vi "FRIC_navX_Internal_SPI_ProcessingLoop.vi"(7 "Device Number":T2, 11 "Rate (4Hz-200Hz)":u8=50 min=4 max=200) -> ()   [LabVIEW 2016]
doc: "This navX VI handles the reading/writing for the navX. All of the good stuff is in here.\nTHIS VI SHOULD NOT BE CALLED BY THE USER!"
uses:
  <vilib>/Rock Robotics/SystemInterfaces/i2clib/i2c_bus.ctl
  TypeDefs/Z900_navX_ProtocolTypeDef.ctl
  navX Library v2.lvlib
  TypeDefs/FRIC_navX_ProcessingLoopStatesTypeDef_I2C.ctl
  TypeDefs/Z900_navX_IntegrationControlRegisters.ctl
  TypeDefs/Z900_navX_ActionTypeDef.ctl
  TypeDefs/Z900_navX_NotifyPacketTypeDef.ctl
  TypeDefs/FRIC_navX_I2C Process Loop TypeDef.ctl
  TypeDefs/Flags/Z900_navX_Flags_CapabilityTypeDef.ctl
  TypeDefs/Z900_navX_DeviceRegisters.ctl
  <vilib>/Rock Robotics/SystemInterfaces/spilib/spi_bus.ctl
  <vilib>/Rock Robotics/WPI/SPI/WPI_SPIDevRef.ctl
  <vilib>/Rock Robotics/WPI/SerialPort/WPI_SerialPortRef.ctl
  TypeDefs/Z900_navX_SerialStreamTypeDef.ctl
  TypeDefs/FRIC_navX_DeviceNumbersTypeDef.ctl
  <vilib>/Rock Robotics/WPI/SerialPort/WPI_SerialPort.ctl
  <vilib>/Platform/TimedLoop/XDataNode/XDataNode.xnode
  <vilib>/Platform/TimedLoop/XDataNode/nitl_modes.ctl
  <vilib>/Platform/TimedLoop/XDataNode/XDNodeRunTimeDep.lvlib
  <vilib>/Platform/TimedLoop/XDataNode/wakeup.ctl
  <vilib>/Platform/TimedLoop/XDataNode/timing_clust.ctl
  <vilib>/ptbypt/NI_PtbyPt.lvlib
  TypeDefs/Z900_navX_DeviceTypeDef.ctl
panel:
  in  "Tab Control":enum32{"Page 1", "Page 2"}(tab)
  in  "Halt":bool
  out "Connected":bool
  in  "SPI Bus":T1=enum."SPI MXP"
  in  "Clock Rate (Hz)":dbl=2000000.0 format="%_6f"
  out "error":errorcluster
  out "Delay":dbl
  out "Loop Time":dbl format="%0.2f"
  out "Loop dt":i64
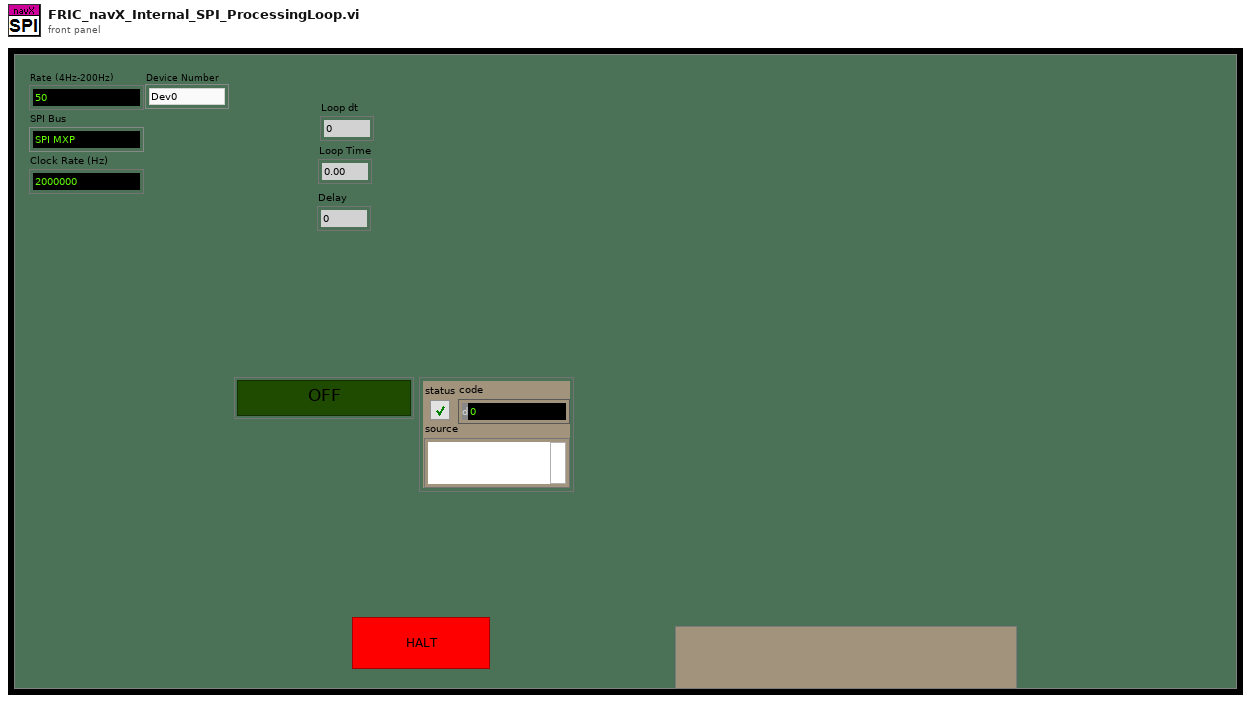
[diagram p1: front panel]
types:
  T1 = typedef "spi_bus.ctl" = enum16{"SPI On-Board, CS0", "SPI On-Board, CS1", "SPI On-Board, CS2", "SPI On-Board, CS3", "SPI MXP", "Invalid"}
  T2 = typedef "FRIC_navX_DeviceNumbersTypeDef.ctl" = enum16{"Dev0", "Dev1", "Dev2", "Dev3"}
  T3 = typedef "FRIC_navX_I2C Process Loop TypeDef.ctl" = cluster{"State Array":T4[], "error":errorcluster, "FPGA Cluster":cluster{"Last Valid FPGA Time":dbl, "Error Count":i32, "Initialized":bool}, "Device Info":T5, "I2CDevRef":cluster{"DevStatus":errorcluster, "Device Address":u8, "Handle":i32, "I2C Bus":T7}, "Registry":u8[], "Command Array":T8[], "Connected?":bool, "navX Device Memory Size":i32, "notification":T9, "Memory Size Set":bool, "SPIDevRef":T11, "navX Serial Open":cluster{"Stream Type":T12, "Serial Port":T13}, "SerialPortRef":T14, "Serial Read Buffer":string, "Serial Write Buffer":string[], "Device Number":T2, "navX SPI Open":cluster{"SPI Bus":T1, "Clock Rate (Hz)":dbl}, "Loop dt":i64, "current time":timestamp, "Loop Time":i64}
  T4 = typedef "FRIC_navX_ProcessingLoopStatesTypeDef_I2C.ctl" = enum16{"Process", "INI", "Check Packets Valid", "Close", "Flush Serial", "Generate Command", "Last Packet Valid", "Open", "Read", "Reset Serial", "Set Termination Char", "Update AE", "Wait", "Write", "Exit"}
  T5 = typedef "navX Library v2.lvlib/Z900_navX_DeviceTypeDef.ctl" = cluster{"Interface":cluster{"Protocol":T6, "Update Rate (4Hz-100Hz)":u8, "navX Open TypeDef":variant}, "Notify Packet":refnum<notifier>, "Loop VI Refnum":refnum<vi>, "Ready to Close Occurrence Refnum":refnum<k4>}
  T6 = typedef "navX Library v2.lvlib/Z900_navX_ProtocolTypeDef.ctl" = enum16{"SERIAL", "I2C", "SPI"}
  T7 = typedef "i2c_bus.ctl" = enum16{"I2C On-Board", "I2C MXP", "Invalid"}
  T8 = typedef "navX Library v2.lvlib/Z900_navX_IntegrationControlRegisters.ctl" = u8
  T9 = typedef "navX Library v2.lvlib/Z900_navX_NotifyPacketTypeDef.ctl" = cluster{"navX Action":T10, "Data":variant}
  T10 = typedef "navX Library v2.lvlib/Z900_navX_ActionTypeDef.ctl" = enum16{"None", "Halt", "Update Serial Protocol", "Zero-Yaw", "Zero-Displacement", "Zero-Velocity"}
  T11 = typedef "WPI_SPIDevRef.ctl" = cluster{"DevStatus":errorcluster, "Handle":i32, "SPI Bus":T1}
  T12 = typedef "navX Library v2.lvlib/Z900_navX_SerialStreamTypeDef.ctl" = enum16{"YRPH", "Quaterinons", "Gyro/Raw", "AHRS", "AHRSAndPositioning"}
  T13 = typedef "WPI_SerialPort.ctl" = enum16{"Onboard RS-232", "MXP TTL", "USB 1", "USB 2"}
  T14 = typedef "WPI_SerialPortRef.ctl" = cluster{"DevStatus":errorcluster, "Serial Port Name":refnum<visa-resource-name>}
  T15 = typedef "XDNodeRunTimeDep.lvlib/timing_clust.ctl" = cluster{"Expected End [f-1]":u64, "Actual End [f-1]":u64, "Finished Late? [f-1]":bool, "Expected End [i-1]":u64, "Actual End [i-1]":u64, "Finished Late? [i-1]":bool, "Expected Start [i]":u64, "Actual Start [i]":u64, "Expected Start [f]":u64, "Actual Start [f]":u64, "Source Name":string, "Structure Name":string, "Period":i64, "Deadline":i64, "Offset":i64, "Start":i64, "Priority":i32, "Timeout":i32, "Mode":T16, "Wakeup Reason":T17, "Error":errorcluster, "Source Type":string, "Secondary Source Type":string, "Global End Time":u64, "Global Start Time":u64, "Frame Duration":u64, "Iteration Duration":u64, "Assigned CPU":i32, "I/O Scan Engine Mode":u32}
  T16 = typedef "XDNodeRunTimeDep.lvlib/nitl_modes.ctl" = enum32{"No Change", "Process missed periods, maintain original phase", "Discard missed periods, maintain original phase", "Process missed periods, ignore original phase", "Discard missed periods, ignore original phase"}
  T17 = typedef "XDNodeRunTimeDep.lvlib/wakeup.ctl" = enum32{"Normal", "Aborted", "Asynchronous wakeup", "Timing source error", "Timed loop error", "Timeout"}
  T18 = typedef "Z900_navX_ActionTypeDef.ctl" = enum16{"None", "Halt", "Normal Read", "Update Serial Protocol", "Update Rate Htz", "Zero-Yaw", "Zero-Displacement", "Zero-Velocity"}
  T19 = typedef "navX Library v2.lvlib/Z900_navX_DeviceRegisters.ctl" = u8
  T20 = typedef "navX Library v2.lvlib/Z900_navX_Flags_CapabilityTypeDef.ctl" = u16
  T21 = cluster{"Last Valid FPGA Time":dbl, "Error Count":i32, "Initialized":bool}
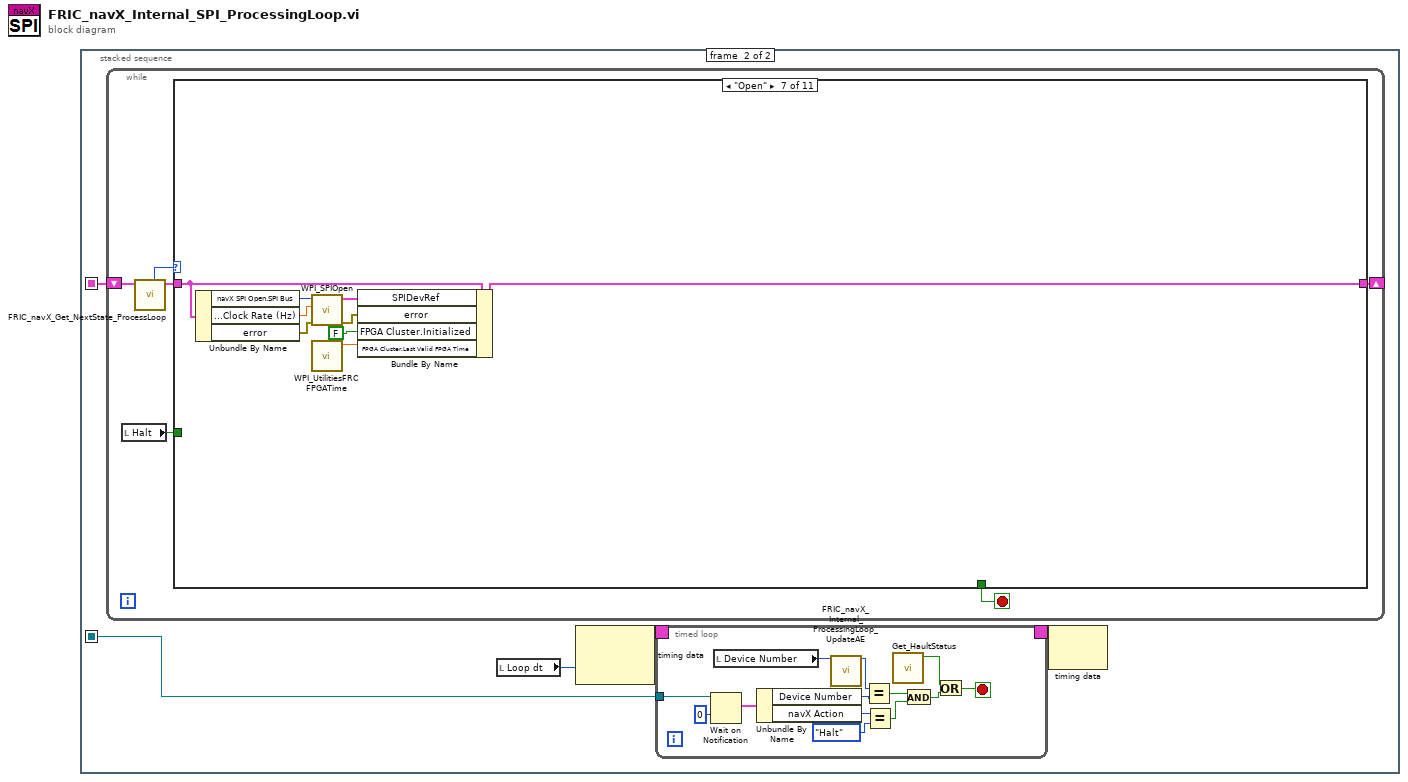
[diagram p0: block diagram]
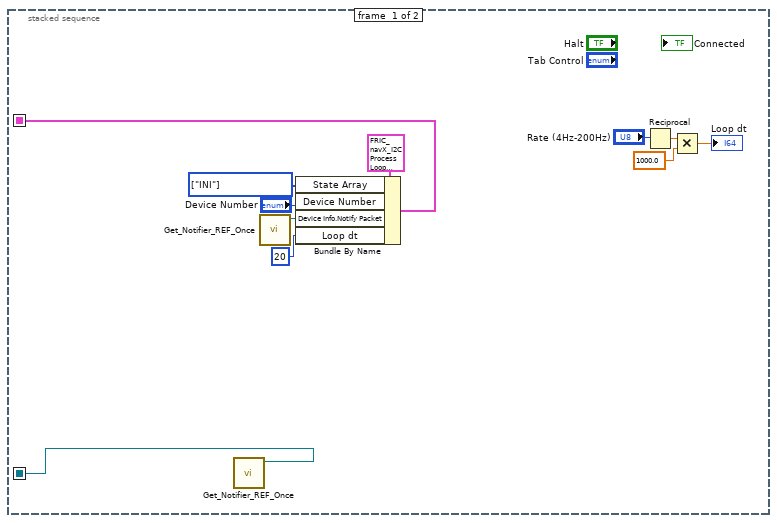
[diagram p2: hidden frame]
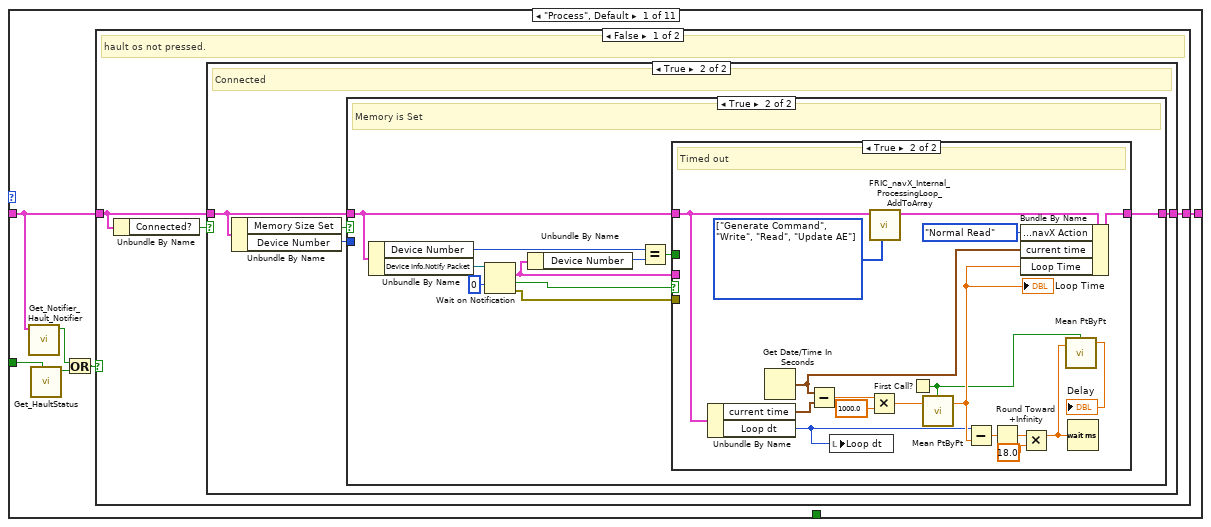
[diagram p3: hidden frame]
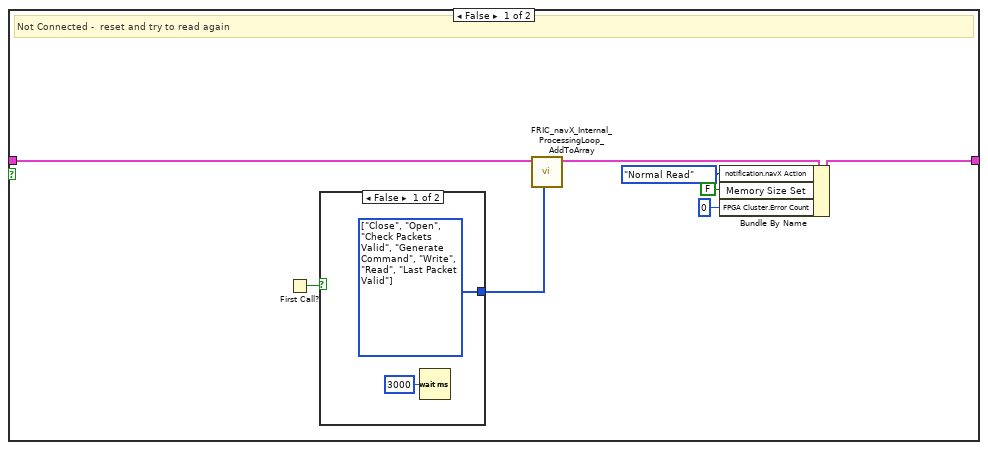
[diagram p4: hidden frame]
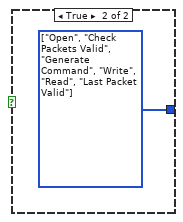
[diagram p5: hidden frame]
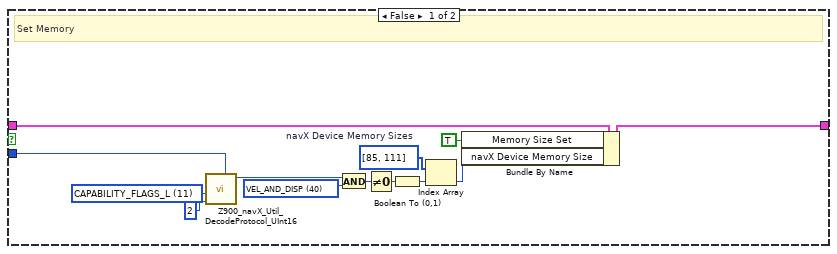
[diagram p6: hidden frame]
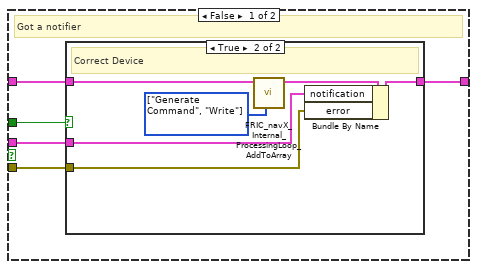
[diagram p7: hidden frame]
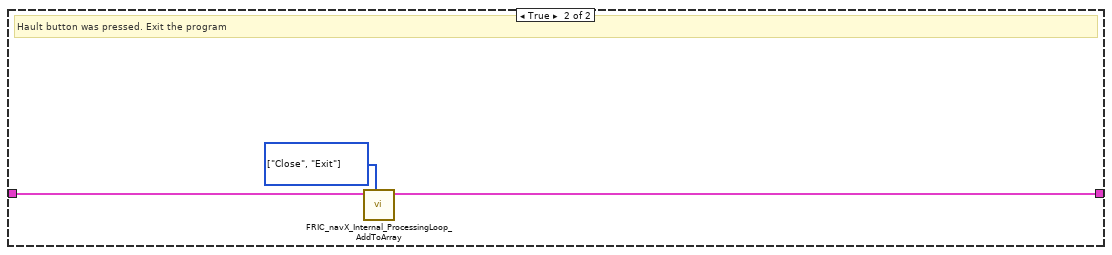
[diagram p9: hidden frame]
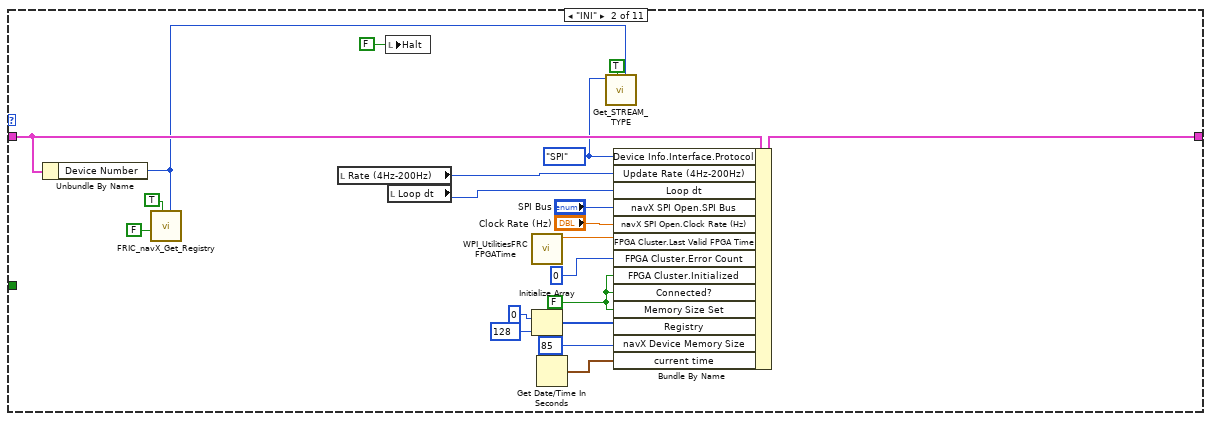
[diagram p10: hidden frame]
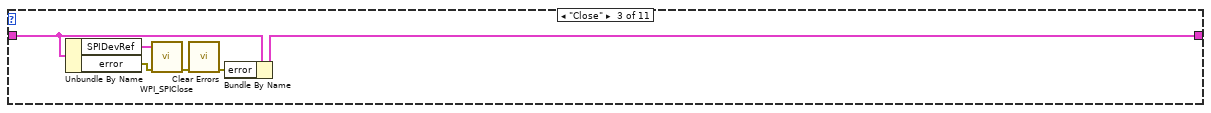
[diagram p11: hidden frame]
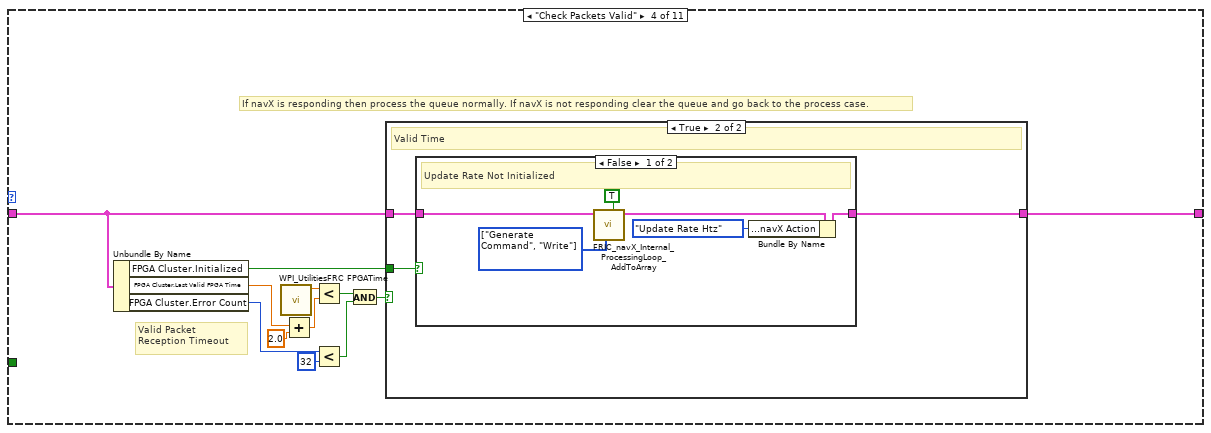
[diagram p12: hidden frame]
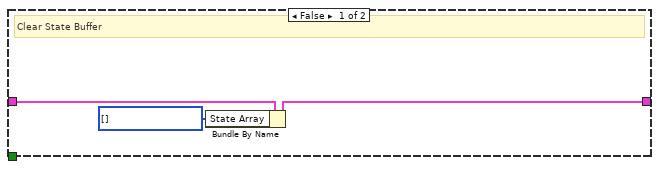
[diagram p13: hidden frame]
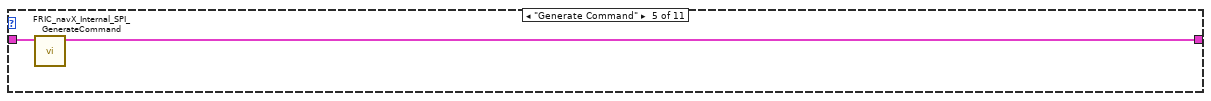
[diagram p15: hidden frame]
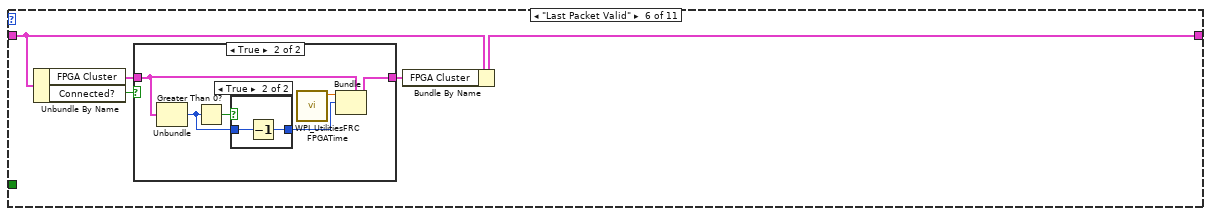
[diagram p16: hidden frame]
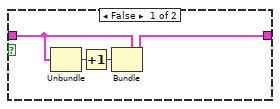
[diagram p17: hidden frame]
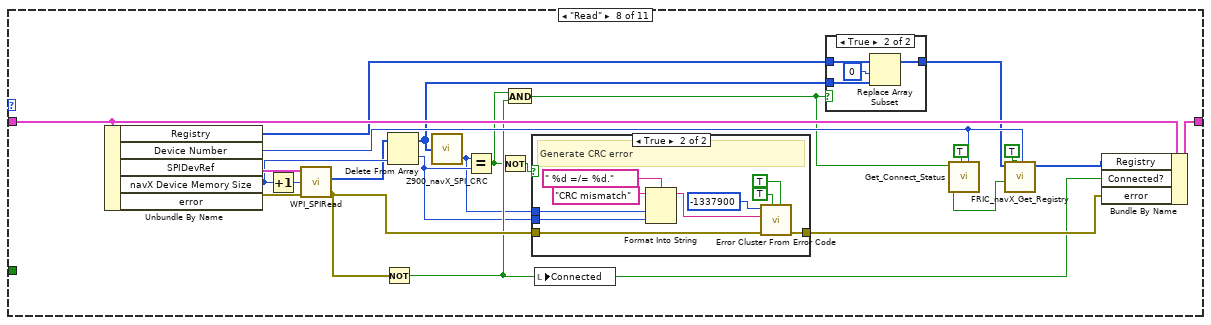
[diagram p19: hidden frame]
diagram:
  n1 = stacked-sequence {
    seq-local: [w11 _] -> [_ w16]
    seq-local: [w5 _] -> [_ w15]
    frame #0 {
      w9 = T4[] [enum."INI"] items=["Process", "INI", "Check Packets Valid", "Close", "Flush Serial", "Generate Command", "Last Packet Valid", "Open", "Read", "Reset Serial", "Set Termination Char", "Update AE", "Wait", "Write", "Exit"] ("State Array")
      n2 = call "Get_Notifier_REF_Once.vi"() -> ("notifier ref out"=w5:refnum<notifier>)  [unwired: 10 in, 1 out]
      n3 = call "Get_Notifier_REF_Once.vi"() -> ("notifier ref out"=w7:refnum<notifier>)  [unwired: 10 in, 1 out]
      n4 = Bundle By Name(cluster=T3 {"State Array"=[enum."INI", enum."Open"], "error"={"status"=FALSE, "code"=0, "source"=""}, "FPGA Cluster"={"Last Valid FPGA Time"=0.0, "Error Count"=0, "Initialized"=FALSE}, "Device Info"={"Interface"={"Protocol"=enum."SERIAL", "Update Rate (4Hz-100Hz)"=4, "navX Open TypeDef"=variant}, "Notify Packet"=refnum, "Loop VI Refnum"=refnum, "Ready to Close Occurrence Refnum"=refnum}, "I2CDevRef"={"DevStatus"={"status"=FALSE, "code"=0, "source"=""}, "Device Address"=0, "Handle"=0, "I2C Bus"=enum."Invalid"}, "Registry"=[], "Command Array"=[214, 32], "Connected?"=FALSE, "navX Device Memory Size"=85, "notification"={"navX Action"=enum."None", "Data"=variant}, "Memory Size Set"=FALSE, "SPIDevRef"={"DevStatus"={"status"=FALSE, "code"=0, "source"=""}, "Handle"=0, "SPI Bus"=enum."SPI On-Board, CS0"}, "navX Serial Open"={"Stream Type"=enum."YRPH", "Serial Port"=enum."Onboard RS-232"}, "SerialPortRef"={"DevStatus"={"status"=FALSE, "code"=0, "source"=""}, "Serial Port Name"=""}, "Serial Read Buffer"="", "Serial Write Buffer"=[], "Device Number"=enum."Dev0", "navX SPI Open"={"SPI Bus"=enum."SPI MXP", "Clock Rate (Hz)"=500000.0}, "Loop dt"=0, "current time"=timestamp(0 s since 1904-01-01), "Loop Time"=0} ("I2C Process Loop TypeDef"), "State Array"=w9, "Device Number"="Device Number", "Device Info.Notify Packet"=w7, "Loop dt"=i64 20) -> (w11:T3)
      n5 = Reciprocal(x="Rate (4Hz-200Hz)") -> (1/x=w2:dbl)
      n6 = Multiply(x=w2, y=1000.0) -> (x*y=→"Loop dt":dbl)
    }
    frame #1 {
      n7 = while {
        shift-right: [w36] -> _
        shift-left: w16 -> [w39]
        stop <- w40 stop-if-true
        n8 = local read "Halt"() -> (w35:bool)
        n9 = call "FRIC_navX_Get_NextState_ProcessLoop.vi"("I2C Process Loop TypeDef (in)"=w39) -> ("I2C Process Loop TypeDef (out)"=w38:T3, "Current State"=w37:T4)  [unwired: 9 in]
        n10 = case shown="\"Open\"" w37 {
          tunnel: [_ _ _ _ _ _ _ _ _ w249 _] -> w40
          tunnel: w38 -> [w45 w129 w146 w150 w173 w177 w200 w222 w246 w251 w259]
          tunnel: [w46 w135 w145 w151 w172 w176 w199 w221 w239 w251 w259] -> w36
          tunnel: w35 -> [w43 _ _ _ _ _ _ _ _ _ _]
          frame "Process", Default {
            n11 = call "Get_Notifier_Hault_Notifier.vi"("Process Loop TypeDef (in)"=w45) -> ("Hault Notifier"=w41:bool)  [unwired: 10 in]
            n12 = call "Get_HaultStatus.vi"("Update"=w43) -> ("Hault"=w42:bool)  [unwired: 10 in]
            n13 = Or(x=w41, y=w42) -> (x .or. y?=w44:bool)
            n14 = case shown="False" w44 {
              tunnel: [w49 w119] -> w46
              tunnel: w45 -> [w47 w120]
              frame False {
                # "hault os not pressed."
                n15 = Unbundle By Name(w47) -> ("Connected?"=w48:bool)
                n16 = case shown="True" w48 {
                  tunnel: w47 -> [w57 w63]
                  tunnel: [w54 w64] -> w49
                  frame False {
                    # "Not Connected -  reset and try to read again"
                    n17 = First Call?() -> (First Call?: T/F=w50:bool)
                    n18 = case shown="False" w50 {
                      tunnel: [w59 w60] -> w56
                      frame False {
                        w59 = T4[] [enum."Close", enum."Open", enum."Check Packets Valid", enum."Generate Command", enum."Write", enum."Read", enum."Last Packet Valid"] items=["Process", "INI", "Check Packets Valid", "Close", "Flush Serial", "Generate Command", "Last Packet Valid", "Open", "Read", "Reset Serial", "Set Termination Char", "Update AE", "Wait", "Write", "Exit"]
                        n19 = Wait (ms)(milliseconds to wait=u32 3000) -> ()  [unwired: 1 out]
                      }
                      frame True {
                        w60 = T4[] [enum."Open", enum."Check Packets Valid", enum."Generate Command", enum."Write", enum."Read", enum."Last Packet Valid"] items=["Process", "INI", "Check Packets Valid", "Close", "Flush Serial", "Generate Command", "Last Packet Valid", "Open", "Read", "Reset Serial", "Set Termination Char", "Update AE", "Wait", "Write", "Exit"]
                      }
                    }
                    n20 = call "FRIC_navX_Internal_ProcessingLoop_AddToArray.vi"("States Array"=w56, "I2C Process Loop TypeDef (in)"=w57) -> ("I2C Process Loop TypeDef (out)"=w55:T3)  [unwired: 9 in]
                    n21 = Bundle By Name(cluster=w55, "notification.navX Action"=Z900_navX_ActionTypeDef."Normal Read", "Memory Size Set"=FALSE, "FPGA Cluster.Error Count"=0) -> (w54:T3)
                  }
                  frame True {
                    # "Connected"
                    n22 = Unbundle By Name(w63) -> ("Memory Size Set"=w62:bool, "Device Number"=w61:T2)
                    n23 = case shown="True" w62 {
                      tunnel: [w76 w85] -> w64
                      tunnel: w63 -> [w77 w83]
                      tunnel: w61 -> [w65 _]
                      frame False {
                        w75 = T19 11 items=["WHOAMI"=0, "HW_REV"=1, "FW_VER_MAJOR"=2, "FW_VER_MINOR"=3, "UPDATE_RATE_HZ"=4, "ACCEL_FSR_G"=5, "GYRO_FSR_DPS"=6, "OP_STATUS"=8, "CAL_STATUS"=9, "SELFTEST_STATUS"=10, "CAPABILITY_FLAGS_L"=11, "CAPABILITY_FLAGS_H"=12, "SENSOR_STATUS"=16, "TIMESTAMP"=18, "YAW"=22, "ROLL"=24, "PITCH"=26, "HEADING"=28, "FUSED_HEADING"=30, "ALTITUDE_I"=32, "ALTITUDE_D"=34, "LINERA_ACC_X"=36, "LINERA_ACC_Y"=38, "LINERA_ACC_Z"=40, "QUAT_W"=42, "QUAT_X"=44, "QUAT_Y"=46, "QUAT_Z"=48, "MPU_TEMP_C"=50, "GYRO_X"=52, "GYRO_Y"=54, "GYRO_Z"=56, "ACC_X"=58, "ACC_Y"=60, "ACC_Z"=62, "MAG_X"=64, "MAG_Y"=66, "MAG_Z"=68, "PRESSURE_I"=70, "PRESSURE_D"=72, "PRESSURE_TEMP"=74, "YAW_OFFSET"=76, "QUAT_OFFSET_W"=78, "QUAT_OFFSET_X"=80, "QUAT_OFFSET_Y"=82, "QUAT_OFFSET_Z"=84, "INTEGRATION_CONTROL"=86, "VELOCITY_X"=88, "VELOCITY_Y"=92, "VELOCITY_Z"=96, "DISPLACMENT_X"=100, "DISPLACMENT_Y"=104, "DISPLACEMENT_Z"=108] ("Device Register")
                        w70 = T20 40 items=["OMNIMOUNT"=4, "OMNIMOUNT_CONFIG_MASK"=38, "VEL_AND_DISP"=40, "YAW_RESET"=80] ("Capability Flag")
                        w71 = i32[] [85, 111]  # navX Device Memory Sizes
                        # "Set Memory"
                        n24 = call "Z900_navX_Util_DecodeProtocol_UInt16.vi"("Device Number"=w65, "length"=2, "Device Register"=w75) -> ("Value"=w68:u16)  [unwired: 8 in]
                        n25 = And(x=w68, y=w70) -> (x .and. y?=w69:T20)
                        n26 = Not Equal To 0?(x=w69) -> (x != 0?=w72:bool)
                        n27 = Boolean To (0,1)(Boolean=w72) -> (0, 1=w73:i16)
                        n28 = Index Array(array=w71, index=w73) -> (element=w66:i32)
                        n29 = Bundle By Name(cluster=w77, "Memory Size Set"=TRUE, "navX Device Memory Size"=w66) -> (w76:T3)
                      }
                      frame True {
                        # "Memory is Set"
                        n30 = Unbundle By Name(w83) -> ("Device Number"=w80:T2, "Device Info.Notify Packet"=w87:refnum<notifier>)
                        n31 = Wait on Notification(notifier=w87, timeout in ms (-1)=0) -> (notification=w81:T9, timed out?=w82:bool, error out=w84:errorcluster)  [unwired: 2 in, 1 out]
                        n32 = Unbundle By Name(w81) -> ("Device Number"=w79:T2)
                        n33 = Equal?(x=w80, y=w79) -> (x = y?=w78:bool)
                        n34 = case shown="True" w82 {
                          tunnel: w83 -> [w92 w113]
                          tunnel: [w91 w115] -> w85
                          tunnel: w81 -> [w90 _]
                          tunnel: w84 -> [w89 _]
                          tunnel: w78 -> [w88 _]
                          frame False {
                            # "Got a notifier"
                            n35 = case shown="True" w88 {
                              tunnel: w92 -> [w93 w99]
                              tunnel: [w93 w98] -> w91
                              tunnel: w90 -> [_ w97]
                              tunnel: w89 -> [_ w94]
                              frame False {
                              }
                              frame True {
                                w95 = T4[] [enum."Generate Command", enum."Write"] items=["Process", "INI", "Check Packets Valid", "Close", "Flush Serial", "Generate Command", "Last Packet Valid", "Open", "Read", "Reset Serial", "Set Termination Char", "Update AE", "Wait", "Write", "Exit"] ("States Array")
                                # "Correct Device"
                                n36 = call "FRIC_navX_Internal_ProcessingLoop_AddToArray.vi"("States Array"=w95, "I2C Process Loop TypeDef (in)"=w99) -> ("I2C Process Loop TypeDef (out)"=w96:T3)  [unwired: 9 in]
                                n37 = Bundle By Name(cluster=w96, "notification"=w97, "error"=w94) -> (w98:T3)
                              }
                            }
                          }
                          frame True {
                            w117 = T4[] [enum."Generate Command", enum."Write", enum."Read", enum."Update AE"] items=["Process", "INI", "Check Packets Valid", "Close", "Flush Serial", "Generate Command", "Last Packet Valid", "Open", "Read", "Reset Serial", "Set Termination Char", "Update AE", "Wait", "Write", "Exit"]
                            # "Timed out"
                            n38 = Unbundle By Name(w113) -> ("current time"=w112:timestamp, "Loop dt"=w100:i64)
                            n39 = Get Date/Time In Seconds() -> (seconds since 1Jan1904=w111:timestamp)
                            n40 = Subtract(x=w111, y=w112) -> (x-y=w110:dbl)
                            n41 = local write "Loop dt"(w100) -> ()
                            n42 = Multiply(x=w110, y=1000.0) -> (x*y=w107:dbl)
                            n43 = call "FRIC_navX_Internal_ProcessingLoop_AddToArray.vi"("States Array"=w117, "I2C Process Loop TypeDef (in)"=w113) -> ("I2C Process Loop TypeDef (out)"=w116:T3)  [unwired: 9 in]
                            n44 = First Call?() -> (First Call?: T/F=w101:bool)
                            n45 = call <vilib>:"Mean PtByPt.vi"("x"=w107, "initialize"=w101) -> ("mean"=w106:dbl)  [unwired: 2 in, 1 out]
                            "Loop Time" <- w106
                            n46 = Subtract(x=w100, y=w106) -> (x-y=w108:dbl)
                            n47 = Round Toward +Infinity(x=w108) -> (ceil(x): smallest int >= x=w104:dbl)
                            n48 = Bundle By Name(cluster=w116, "notification.navX Action"=Z900_navX_ActionTypeDef."Normal Read", "current time"=w111, "Loop Time"=w106) -> (w115:T3)
                            n49 = Multiply(x=w104, y=18.0) -> (x*y=w103:dbl)
                            n50 = call <vilib>:"Mean PtByPt.vi"("x"=w103, "initialize"=w101) -> ("mean"=→"Delay":dbl)  [unwired: 2 in, 1 out]
                            n51 = Wait (ms)(milliseconds to wait=w103) -> ()  [unwired: 1 out]
                          }
                        }
                      }
                    }
                  }
                }
              }
              frame True {
                w118 = T4[] [enum."Close", enum."Exit"] items=["Process", "INI", "Check Packets Valid", "Close", "Flush Serial", "Generate Command", "Last Packet Valid", "Open", "Read", "Reset Serial", "Set Termination Char", "Update AE", "Wait", "Write", "Exit"] ("States Array")
                # "Hault button was pressed. Exit the program"
                n52 = call "FRIC_navX_Internal_ProcessingLoop_AddToArray.vi"("States Array"=w118, "I2C Process Loop TypeDef (in)"=w120) -> ("I2C Process Loop TypeDef (out)"=w119:T3)  [unwired: 9 in]
              }
            }
          }
          frame "INI" {
            w121 = Z900_navX_ProtocolTypeDef."SPI" ("Protocol")
            w133 = FALSE ("Initialized")
            n53 = Unbundle By Name(w129) -> ("Device Number"=w122:T2)
            n54 = call "FRIC_navX_Get_Registry.vi"("Device Number"=w122, "Update"=TRUE, "Connected?"=FALSE) -> ()  [unwired: 7 in, 2 out]
            n55 = local read "Rate (4Hz-200Hz)"() -> (w125:u8)
            n56 = local write "Halt"(FALSE ("Halt")) -> ()
            n57 = local read "Loop dt"() -> (w124:i64)
            n58 = call <vilib>:"WPI_UtilitiesFRC FPGATime.vi"() -> ("FPGA Time"=w137:dbl)  [unwired: 10 in, 1 out]
            n59 = Initialize Array(u8 0 ("Received Data"), 128 ("hex")) -> (w131:u8[])
            n60 = Get Date/Time In Seconds() -> (seconds since 1Jan1904=w126:timestamp)
            n61 = call "Get_STREAM_TYPE.vi"("Device Number"=w122, "Update"=TRUE, "Protocol (in)"=w121) -> ()  [unwired: 8 in, 1 out]
            n62 = Bundle By Name(cluster=w129, "Device Info.Interface.Protocol"=w121, "Update Rate (4Hz-200Hz)"=w125, "Loop dt"=w124, "navX SPI Open.SPI Bus"="SPI Bus", "navX SPI Open.Clock Rate (Hz)"="Clock Rate (Hz)", "FPGA Cluster.Last Valid FPGA Time"=w137, "FPGA Cluster.Error Count"=0 ("Error Count"), "FPGA Cluster.Initialized"=w133, "Connected?"=w133, "Memory Size Set"=w133, "Registry"=w131, "navX Device Memory Size"=85 ("hex"), "current time"=w126) -> (w135:T3)
          }
          frame "Close" {
            n63 = Unbundle By Name(w146) -> ("SPIDevRef"=w144:T11, "error"=w143:errorcluster)
            n64 = call <vilib>:"WPI_SPIClose.vi"("error in (no error)"=w143, "SPIDevRef"=w144) -> ("error out"=w142:errorcluster)  [unwired: 9 in]
            n65 = call <vilib>:"Clear Errors.vi"("error in (no error)"=w142) -> ("error out"=w141:errorcluster)  [unwired: 5 in, 1 out]
            n66 = Bundle By Name(cluster=w146, "error"=w141) -> (w145:T3)
          }
          frame "Check Packets Valid" {
            # "If navX is responding then process the queue normally. If navX is not responding clear the queue and go back to the process case."
            # "Valid Packet Reception Timeout"
            n67 = Unbundle By Name(w150) -> ("FPGA Cluster.Initialized"=w148:bool, "FPGA Cluster.Last Valid FPGA Time"=w149:dbl, "FPGA Cluster.Error Count"=w147:i32)
            n68 = call <vilib>:"WPI_UtilitiesFRC FPGATime.vi"() -> ("FPGA Time"=w156:dbl)  [unwired: 10 in, 1 out]
            n69 = Add(x=w149, y=2.0) -> (x+y=w157:dbl)
            n70 = Less?(x=w156, y=w157) -> (x < y?=w154:bool)
            n71 = Less?(x=w147, y=32) -> (x < y?=w153:bool)
            n72 = And(x=w154, y=w153) -> (x .and. y?=w152:bool)
            n73 = case shown="True" w152 {
              tunnel: w150 -> [w161 w164]
              tunnel: [w160 w163] -> w151
              tunnel: w148 -> [_ w162]
              frame False {
                w159 = T4[] [] items=["Process", "INI", "Check Packets Valid", "Close", "Flush Serial", "Generate Command", "Last Packet Valid", "Open", "Read", "Reset Serial", "Set Termination Char", "Update AE", "Wait", "Write", "Exit"] ("f")
                # "Clear State Buffer"
                n74 = Bundle By Name(cluster=w161, "State Array"=w159) -> (w160:T3)
              }
              frame True {
                # "Valid Time"
                n75 = case shown="False" w162 {
                  tunnel: w164 -> [w169 w171]
                  tunnel: [w167 w171] -> w163
                  frame False {
                    w165 = T4[] [enum."Generate Command", enum."Write"] items=["Process", "INI", "Check Packets Valid", "Close", "Flush Serial", "Generate Command", "Last Packet Valid", "Open", "Read", "Reset Serial", "Set Termination Char", "Update AE", "Wait", "Write", "Exit"] ("f")
                    # "Update Rate Not Initialized"
                    n76 = call "FRIC_navX_Internal_ProcessingLoop_AddToArray.vi"("Add to beginning"=TRUE, "States Array"=w165, "I2C Process Loop TypeDef (in)"=w169) -> ("I2C Process Loop TypeDef (out)"=w168:T3)  [unwired: 8 in]
                    n77 = Bundle By Name(cluster=w168, "notification.navX Action"=Z900_navX_ActionTypeDef."Update Rate Htz") -> (w167:T3)
                  }
                  frame True {
                    # "Update Rate is Initialized"
                  }
                }
              }
            }
          }
          frame "Generate Command" {
            n78 = call "FRIC_navX_Internal_SPI_GenerateCommand.vi"("I2C Process Loop TypeDef (in)"=w173) -> ("I2C Process Loop TypeDef (out)"=w172:T3)  [unwired: 10 in]
          }
          frame "Last Packet Valid" {
            n79 = Unbundle By Name(w177) -> ("FPGA Cluster"=w178:T21, "Connected?"=w174:bool)
            n80 = case shown="True" w174 {
              tunnel: [w181 w188] -> w175
              tunnel: w178 -> [w180 w184]
              frame False {
                n81 = Unbundle(w180) -> ("Error Count"=w179:i32)  [unwired: 2 out]
                n82 = Increment(x=w179) -> (x+1=w182:i32)
                n83 = Bundle(cluster=w180, "Error Count"=w182) -> (w181:T21)  [unwired: 2 in]
              }
              frame True {
                n84 = Unbundle(w184) -> ("Error Count"=w183:i32)  [unwired: 2 out]
                n85 = Greater Than 0?(x=w183) -> (x > 0?=w186:bool)
                n86 = case shown="True" w186 {
                  tunnel: [w189 w191] -> w185
                  tunnel: w183 -> [w189 w190]
                  frame False {
                  }
                  frame True {
                    n87 = Decrement(x=w190) -> (x-1=w191:i32)
                  }
                }
                n88 = call <vilib>:"WPI_UtilitiesFRC FPGATime.vi"() -> ("FPGA Time"=w187:dbl)  [unwired: 10 in, 1 out]
                n89 = Bundle(cluster=w184, "Last Valid FPGA Time"=w187, "Error Count"=w185) -> (w188:T21)  [unwired: 1 in]
              }
            }
            n90 = Bundle By Name(cluster=w177, "FPGA Cluster"=w175) -> (w176:T3)
          }
          frame "Open" {
            n91 = Unbundle By Name(w200) -> ("navX SPI Open.SPI Bus"=w193:T1, "navX SPI Open.Clock Rate (Hz)"=w192:dbl, "error"=w194:errorcluster)
            n92 = call <vilib>:"WPI_SPIOpen.vi"("error in"=w194, "Clock Rate (Hz)"=w192, "SPI Bus"=w193) -> ("error out"=w196:errorcluster, "SPIDevRef"=w197:T11)  [unwired: 7 in]
            n93 = call <vilib>:"WPI_UtilitiesFRC FPGATime.vi"() -> ("FPGA Time"=w195:dbl)  [unwired: 10 in, 1 out]
            n94 = Bundle By Name(cluster=w200, "SPIDevRef"=w197, "error"=w196, "FPGA Cluster.Initialized"=FALSE ("Initialized"), "FPGA Cluster.Last Valid FPGA Time"=w195) -> (w199:T3)
          }
          frame "Read" {
            n95 = Unbundle By Name(w222) -> ("Registry"=w219:u8[], "Device Number"=w213:T2, "SPIDevRef"=w218:T11, "navX Device Memory Size"=w215:i32, "error"=w217:errorcluster)
            n96 = Increment(x=w215) -> (x+1=w214:i32)
            n97 = call <vilib>:"WPI_SPIRead.vi"("error in (no error)"=w217, "Num to Read"=w214, "SPIDevRef"=w218) -> ("error out"=w211:errorcluster, "Received Data"=w207:u8[])  [unwired: 6 in, 1 out]
            n98 = Not(x=w211) -> (.not. x?=w210:bool)
            n99 = Delete From Array(array=w207, index=w215) -> (deleted portion=w205:u8, array with subset deleted=w203:u8[])  [unwired: 1 in]
            n100 = call "Z900_navX_SPI_CRC.vi"("Message"=w203) -> ("CRC"=w202:u8)  [unwired: 1 out]
            n101 = Equal?(x=w202, y=w205) -> (x = y?=w206:bool)
            n102 = Not(x=w206) -> (.not. x?=w204:bool)
            n103 = And(x=w206, y=w210) -> (x .and. y?=w208:bool)
            n104 = case shown="True" w204 {
              tunnel: w202 -> [_ w231]
              tunnel: w205 -> [_ w230]
              tunnel: w211 -> [w223 w227]
              tunnel: [w223 w226] -> w216
              frame False {
              }
              frame True {
                # "Generate CRC error"
                n105 = Format Into String(format string=" %d =/= %d.", initial string="CRC mismatch", w231, w230) -> (resulting string=w228:string)  [unwired: 1 in, 1 out]
                n106 = call <vilib>:"Error Cluster From Error Code.vi"("is warning? (False)"=TRUE, "show call chain? (False)"=TRUE, "error in (no error)"=w227, "error message (\"\")"=w228, "error code (0)"=-1337900 ("code")) -> ("error out"=w226:errorcluster)  [unwired: 4 in]
              }
            }
            n107 = local write "Connected"(w210) -> ()
            n108 = case shown="True" w208 {
              tunnel: w219 -> [_ w238]
              tunnel: [w234 w237] -> w201
              tunnel: w203 -> [w234 w236]
              frame False {
              }
              frame True {
                n109 = Replace Array Subset(array=w238, new element=w236, index=u8 0 ("hex")) -> (w237:u8[])
              }
            }
            n110 = call "Get_Connect_Status.vi"("Device Number"=w213, "Update"=TRUE, "Connected"=w208) -> ()  [unwired: 8 in, 1 out]
            n111 = call "FRIC_navX_Get_Registry.vi"("Device Number"=w213, "Update"=TRUE, "Connected?"=w208, "Registry (in)"=w201) -> ("Registry (out)"=w220:u8[])  [unwired: 6 in, 1 out]
            n112 = Bundle By Name(cluster=w222, "Registry"=w220, "Connected?"=w210, "error"=w216) -> (w221:T3)
          }
          frame "Write" {
            n113 = Unbundle By Name(w246) -> ("SPIDevRef"=w245:T11, "Command Array"=w244:T8[], "I2CDevRef.DevStatus"=w243:errorcluster)
            n114 = call <vilib>:"WPI_SPIWrite.vi"("error in (no error)"=w243, "Data To Send"=w244, "SPIDevRef"=w245) -> ("error out"=w242:errorcluster, "SPIDevRef"=w241:T11)  [unwired: 6 in, 1 out]
            n115 = Bundle By Name(cluster=w246, "SPIDevRef"=w241, "error"=w242) -> (w240:T3)
            n116 = flat-sequence {
              tunnel: w240 -> [w248]
              tunnel: [w248] -> w239
              frame #0 {
                n117 = Wait (ms)(milliseconds to wait=u32 1) -> ()  [unwired: 1 out]
              }
            }
          }
          frame "Exit" {
            n118 = Unbundle By Name(w251) -> ("Device Info"=w250:T5)
            n119 = in-place {
              in-place-border: [TRUE] -> w249
              in-place-border: w250 -> [w252]
              # "Set Occurence of Close"
              n120 = Unbundle By Name(w252) -> ("Ready to Close Occurrence Refnum"=w254:refnum<k4>)
              n121 = local write "Halt"(FALSE ("Halt")) -> ()
              n122 = Set Occurrence(w254) -> ()
            }
          }
          frame "Update AE" {
            n123 = Unbundle By Name(w259) -> ("Device Number"=w256:T2, "error"=w258:errorcluster)
            "error" <- w258
            n124 = call "Get_Error_Status.vi"("Device Number"=w256, "Update"=TRUE, "error in"=w258) -> ()  [unwired: 8 in, 1 out]
          }
        }
      }
      n125 = local read "Loop dt"() -> (w12:i64)
      n126 = node-c288(w12) -> (w14:T15)  [unwired: 1 in]
      n127 = timed-loop {
        timing: w14 -> [_]
        timing-out: [_] -> w13
        tunnel: w15 -> [w25]
        stop <- w17 stop-if-true
        n128 = Wait on Notification(notifier=w25, timeout in ms (-1)=0) -> (notification=w24:T9)  [unwired: 2 in, 3 out]
        n129 = local read "Device Number"() -> (w22:T2)
        n130 = Unbundle By Name(w24) -> ("Device Number"=w23:T2, "navX Action"=w27:T10)
        n131 = call "FRIC_navX_Internal_ProcessingLoop_UpdateAE.vi"("Device Number"=w22) -> ()  [unwired: 15 in]
        n132 = Equal?(x=w22, y=w23) -> (x = y?=w21:bool)
        n133 = Equal?(x=w27, y=Z900_navX_ActionTypeDef."Halt") -> (x = y?=w20:bool)
        n134 = call "Get_HaultStatus.vi"() -> ("Hault"=w19:bool)  [unwired: 11 in]
        n135 = And(x=w21, y=w20) -> (x .and. y?=w18:bool)
        n136 = Or(x=w19, y=w18) -> (x .or. y?=w17:bool)
      }
      n137 = node-c288(w13) -> ()  [unwired: 1 out]
    }
  }
